vi "Keep Description.vi"(9 "Same Desc":bool, 10 "Array":i32[](array[numeric]), 11 "Value in":string[](array[string])) -> (3 "Value out":string[](array[string]))   [LabVIEW 2020, in "DocTool.lvlib"]
uses:
  DocTool.lvlib
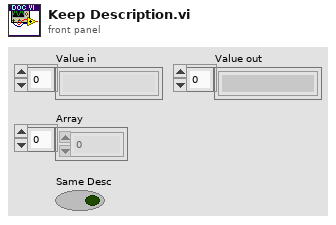
[diagram p1: front panel]
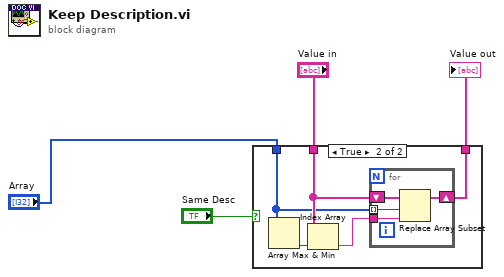
[diagram p0: block diagram]
diagram:
  n1 = case shown="True" "Same Desc" {
    tunnel: "Value in" -> [w5 w10]
    tunnel: "Array" -> [_ w8]
    tunnel: [w5 w7] -> w3
    frame False {
    }
    frame True {
      n2 = Array Max & Min(array=w8) -> (min index (indices)=w6:i32)  [unwired: 3 out]
      n3 = Index Array(array=w10, index=w6) -> (element=w9:string)
      n4 = for {
        tunnel: w9 -> [w13]
        tunnel: w8 -> [w12] mode=indexing
        shift-right: [w11] -> w7
        shift-left: w10 -> [w14]
        n5 = Replace Array Subset(array=w14, new element=w13, index=w12) -> (w11:string[])
      }
    }
  }
  "Value out" <- w3
